vi "ExportContainerContent.vi"(6 "CodeSchema":string, 8 "error in (no error)":errorcluster, 10 "ILabVIEWItem in":refnum<class "ILabVIEWItem.lvclass">, 11 "CGrapherDGML in":refnum<class "CGrapherDGML.lvclass">) -> (0 "error out":errorcluster, 1 "Links":T1, 2 "Nodes":T1, 3 "CGrapherDGML":refnum<class "CGrapherDGML.lvclass">)   [LabVIEW 2020, in "DefaultExtensions.lvlib" / "CGrapherDGML.lvclass"]
uses:
  CGrapherDGML.lvclass
  LabVIEWObjectInterfaces/ILabVIEWItem/ILabVIEWItem.lvclass
  LabVIEWItem/CLabVIEWItem/ConnectionSet.ctl
  CGrapherDGML.lvclass/CGrapherDGML.ctl
  02eefc4a-eede-484c-8d24-8de4f53580c2.vi
  LabVIEWItem/CLabVIEWItem/CLabVIEWItem.lvclass
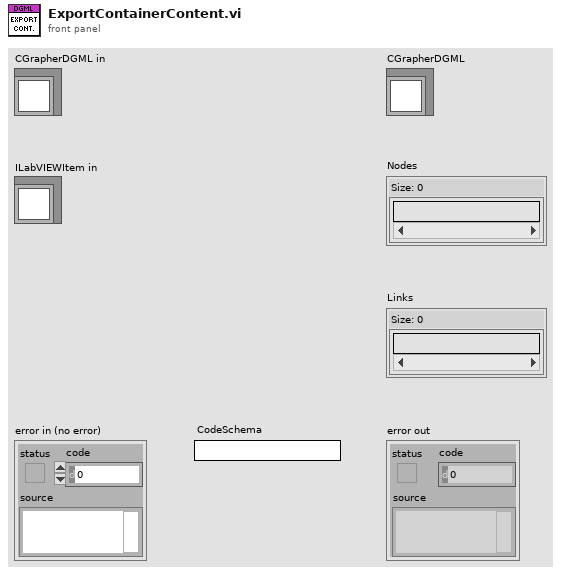
[diagram p1: front panel]
types:
  T1 = typedef "LabVIEWItem.lvlib/CLabVIEWItem.lvclass/ConnectionSet.ctl" = set{string}
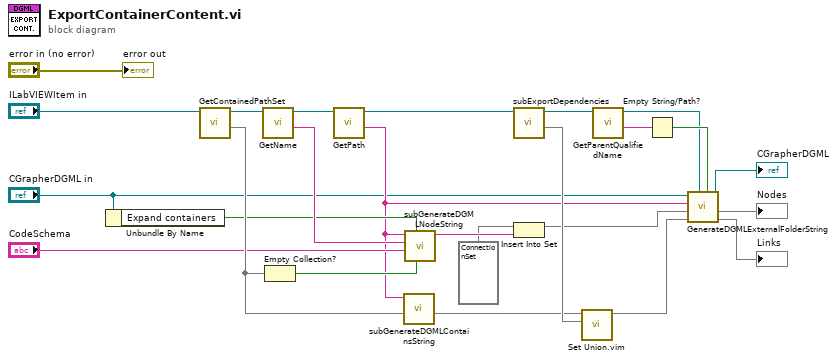
[diagram p0: block diagram]
diagram:
  n1 = Unbundle By Name("CGrapherDGML in") -> ("Expand containers"=w9:bool)
  n2 = call-dynamic "GetContainedPathSet.vi"("ILabVIEWItem in"="ILabVIEWItem in") -> ("Contained"=w13:set{string}, "ILabVIEWItem out"=w11:refnum<class "ILabVIEWItem.lvclass">)  [unwired: 8 in, 1 out]
  n3 = call-dynamic "GetName.vi"("ILabVIEWItem in"=w11) -> ("Name"=w21:string, "ILabVIEWItem out"=w25:refnum<class "ILabVIEWItem.lvclass">)  [unwired: 8 in, 1 out]
  n4 = Empty Collection?(1:w13) -> (0:w20:bool)
  n5 = call-dynamic "GetPath.vi"("ILabVIEWItem in"=w25) -> ("Path"=w6:string, "ILabVIEWItem out"=w23:refnum<class "ILabVIEWItem.lvclass">)  [unwired: 8 in, 1 out]
  n6 = call "subGenerateDGMLContainsString.vi"("Contained"=w13, "Source"=w6) -> ("Links"=w18:T1)  [unwired: 9 in]
  n7 = call "subGenerateDGMLNodeString.vi"("Container empty?"=w20, "Expand?"=w9, "Code schema"="CodeSchema", "Label"=w21, "Id"=w6) -> ("Node string"=w19:string)  [unwired: 6 in]
  n8 = call "subExportDependencies.vi"("ILabVIEWItem in"=w23) -> ("Links"=w22:T1, "ILabVIEWItem out"=w17:refnum<class "ILabVIEWItem.lvclass">)  [unwired: 8 in, 1 out]
  n9 = Insert Into Set(10:w19, 11:T1 {} ("Links")) -> (3:w7:T1)  [unwired: 1 out]
  n10 = call "Set Union.vim"("set 2"=w22, "set 1"=w18) -> ("union"=w8:T1)  [unwired: 9 in]
  n11 = call-dynamic "GetParentQualifiedName.vi"("ILabVIEWItem in"=w17) -> ("Name"=w16:string, "ILabVIEWItem out"=w3:refnum<class "ILabVIEWItem.lvclass">)  [unwired: 8 in, 1 out]
  n12 = Empty String/Path?(string/path=w16) -> (empty?=w15:bool)
  n13 = call-dynamic "GenerateDGMLExternalFolderString.vi"("Apply? (T)"=w15, "ILabVIEWItem in"=w3, "Links in"=w8, "Nodes in"=w7, "Path in"=w6, "CGrapherDGML in"="CGrapherDGML in") -> ("Links"=→"Links":T1, "Nodes"=→"Nodes":T1, "CGrapherDGML"=→"CGrapherDGML":refnum<class "CGrapherDGML.lvclass">)  [unwired: 3 in]
  "error out" <- "error in (no error)"
